vi "Subtractor0.vi"() -> (8 "Subtractor0":refnum<class "Subtractor0.lvclass">)   [LabVIEW 2017, in "Subtractor0.lvclass"]
uses:
  Subtractor0.lvclass
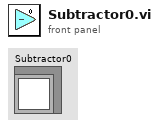
[diagram p1: front panel]
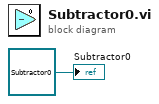
[diagram p0: block diagram]
diagram:
  "Subtractor0" <- refnum<class "Subtractor0.lvclass"> refnum ("Subtractor0.lvclass")
